vi "getSampleRate_6229.vi"(1 "Number of active channels":i32) -> (0 "Sample Rate":dbl=1000000.0)   [LabVIEW 2016]
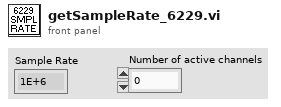
[diagram p1: front panel]
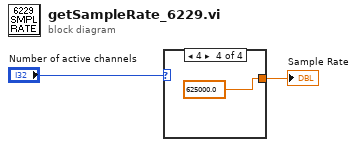
[diagram p0: block diagram]
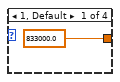
[diagram p2: hidden frame]
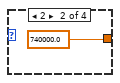
[diagram p3: hidden frame]
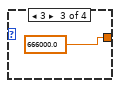
[diagram p4: hidden frame]
diagram:
  n1 = case shown="4" "Number of active channels" {
    tunnel: [833000.0 740000.0 666000.0 625000.0] -> w1
    frame 1, Default {
    }
    frame 2 {
    }
    frame 3 {
    }
    frame 4 {
    }
  }
  "Sample Rate" <- w1
